vi "fgt set manual.vi"(8 "error in (no error)":errorcluster, 10 "value":sgl=5.0, 11 "pressureIndex":u32) -> (0 "error out":errorcluster)   [LabVIEW 2016, in "fgt_SDK.lvlib"]
doc: "Manually set internal solenoid valve voltage. This stops pressure regulation on the channel until a new pressure or flow rate command is set."
uses:
  fgt_SDK.lvlib
  dlls/fgt_SDK_32.dll
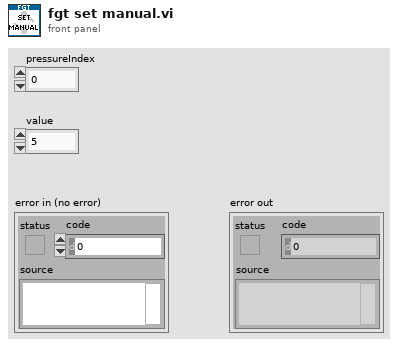
[diagram p1: front panel]
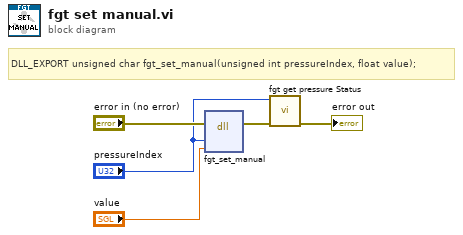
[diagram p0: block diagram]
diagram:
  # "DLL_EXPORT unsigned char fgt_set_manual(unsigned int pressureIndex, float value);"
  n1 = dll-call lib="C:/projects/SDK/fgt-sdk-labview/dlls/fgt_SDK_*.*" fn="fgt_set_manual"(error in="error in (no error)", "pressureIndex"="pressureIndex", "value"="value") -> (error out=w3:errorcluster)  [unwired: 5 in, 1 out]
  n2 = call "fgt get pressure Status.vi"("error in (no error)"=w3, "pressureIndex"="pressureIndex") -> ("error out"=→"error out":errorcluster)  [unwired: 9 in]
